vi "pause after every move.vi"(1 "next action in":T1) -> (0 "next action out":T1)   [LabVIEW 2020, in "core.lvlib"]
uses:
  core.lvlib
  action.ctl
  pause after every move (global variable).vi
  pause (global variable).vi
  main/main.lvlib
panel:
  # "Development\ncontrols/indicators useful for development and testing, but which are not outputs of the VI"
  # "Input\nInputs to the VI"
  # "Output\nOutputs of the VI"
  # "Description\n\nBlank VI with error handling case. \n\nSummarize the use of this VI in this space."
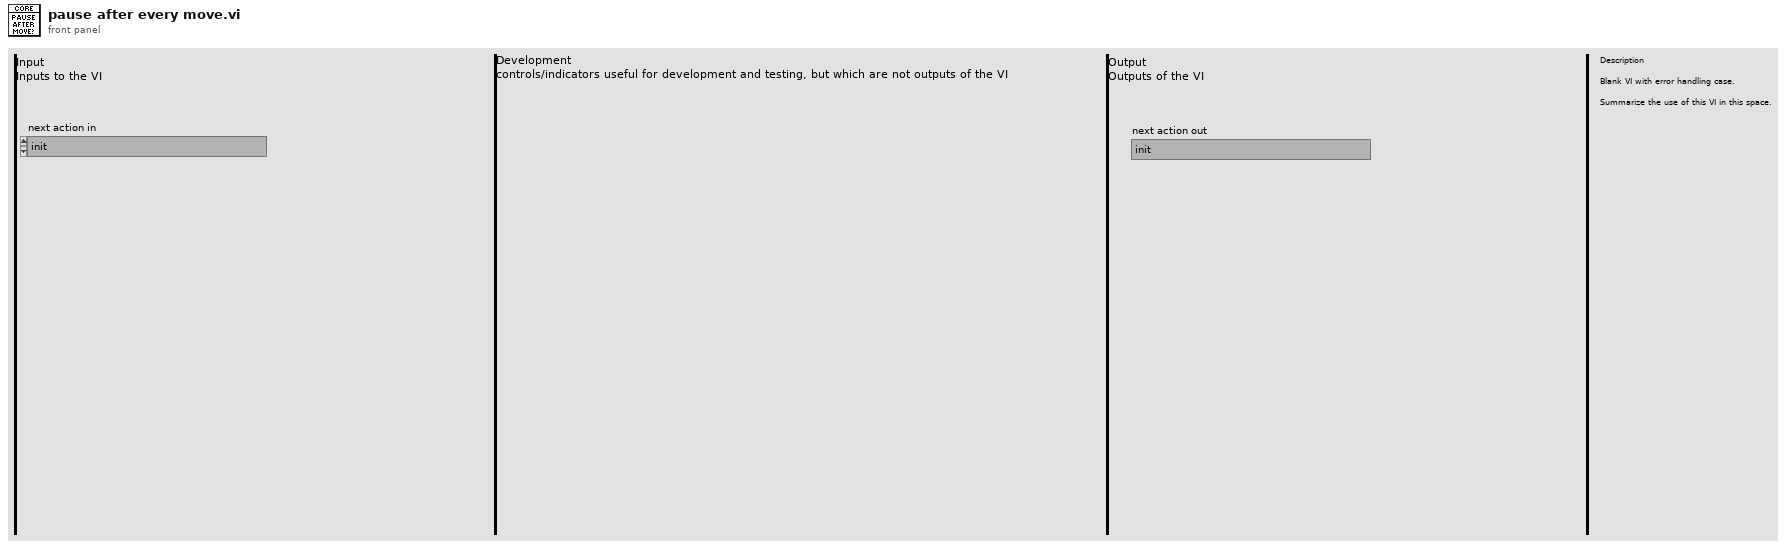
[diagram p1: front panel]
types:
  T1 = typedef "core.lvlib/action.ctl" = enum16{"init", "move_forward", "move_backward", "complete_tour", "exit", "be idle (do nothing)"}
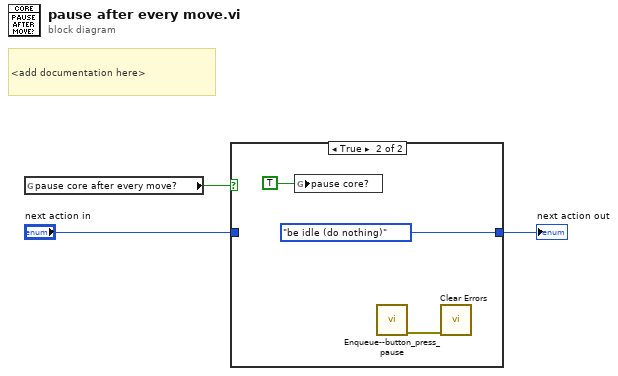
[diagram p0: block diagram]
diagram:
  # "<add documentation here>"
  n1 = global read "pause after every move (global variable).vi" "pause core after every move?"() -> (w3:bool)
  n2 = case shown="True" w3 {
    tunnel: "next action in" -> [w4 _]
    tunnel: [w4 action."be idle (do nothing)" ("next action in")] -> w1
    frame False {
    }
    frame True {
      n3 = global write "pause (global variable).vi" "pause core?"(TRUE ("pause core?")) -> ()
      n4 = call "Enqueue--button_press_pause.vi"() -> ("error out"=w5:errorcluster)  [unwired: 11 in]
      n5 = call <vilib>:"Clear Errors.vi"("error in (no error)"=w5) -> ()  [unwired: 5 in, 2 out]
    }
  }
  "next action out" <- w1
